vi "Create FPGA Addon.vi"(7 "group scalars":bool, 8 "error in":errorcluster, 10 "FPGA addon name":string, 11 "target in":refnum<k39>) -> (0 "error out":errorcluster, 2 "FPGA addon refnum":T1=18446744073709551615 format="%.0x", 3 "target out":refnum<k39>)   [LabVIEW 2026, in "Scripting API.lvlib"]
doc: "Creates an FPGA addon custom device within the provided System Definition Target. The FPGA addon name must be unique, otherwise the VI will return an error. The VI returns the reference of the created custom device.\n\nIf set to \"True\", the \"group scalars\" option allows the custom device to organize the FPGA bitfile controls and indicators into a folder structure following the \".\" notation (i.e. control bitfile name -> \"Group.myControl\" becomes a system definition channel \"myControl\" in the \"Group\" section -> Group\\myControl)"
uses:
  Scripting API.lvlib
  C:/Users/Administrator/Desktop/Jatin/All DNC DLLs/NationalInstruments.VeriStand.SystemDefinitionAPI.dll
  Jatin/All DNC DLLs/NationalInstruments.VeriStand.SystemDefinitionAPI.dll
  <vilib>/NI VeriStand/Custom Device API/Custom Device Item Ref.ctl
  Addon/Addon Shared/Types/FG Action.ctl
  Addon/Addon Shared/Types/FPGA Settings.ctl
  Addon/Addon Shared/SubVIs/Constants.vi
  <vilib>/NI VeriStand/Custom Device API/NI VeriStand - Get Item Property.vi
  <vilib>/NI VeriStand/Custom Device API/Get Item Property (Path).vi
  <vilib>/NI VeriStand/Custom Device API/Get Item Property (String).vi
  <vilib>/NI VeriStand/Custom Device API/Get Item Property (Boolean).vi
  <vilib>/NI VeriStand/Custom Device API/NI VeriStand - Set Item Property.vi
  <vilib>/NI VeriStand/Custom Device API/Set Item Property (Path).vi
  <vilib>/NI VeriStand/Custom Device API/Set Item Property (String).vi
  <vilib>/NI VeriStand/Custom Device API/Set Item Property (Boolean).vi
  Addon/Addon Shared/FPGA Addon Shared.lvlib
  <vilib>/NI VeriStand/Custom Device API/Custom Device API.lvlib
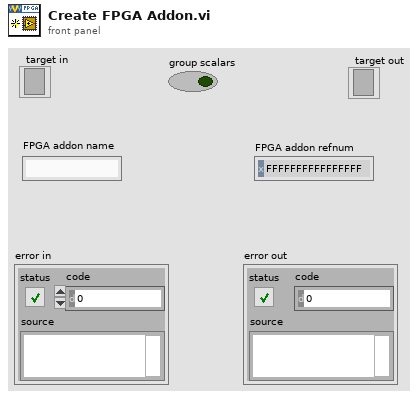
[diagram p1: front panel]
types:
  T1 = typedef "Custom Device API.lvlib/Custom Device Item Ref.ctl" = u64
  T2 = typedef "FPGA Addon Shared.lvlib/FPGA Settings.ctl" = cluster{"Bitfile path":path, "RIO Device Address":string, "Group":bool}
  T3 = typedef "FPGA Addon Shared.lvlib/FG Action.ctl" = enum8{"GET", "SET"}
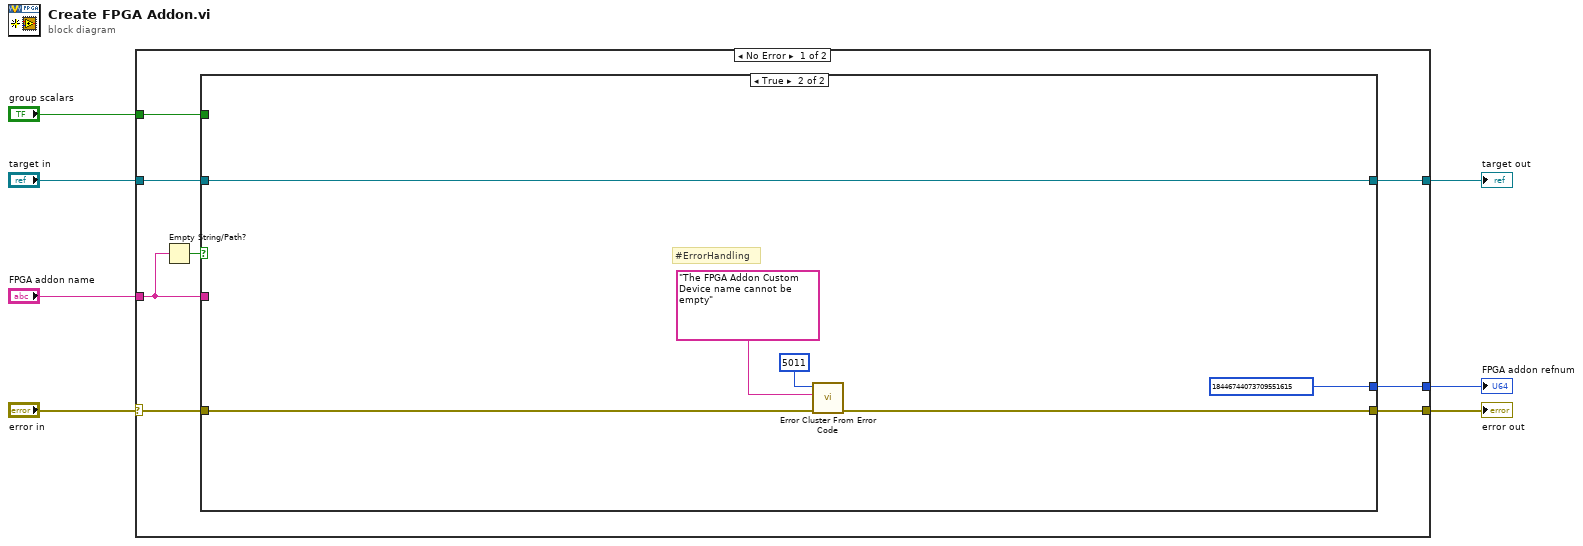
[diagram p0: block diagram]
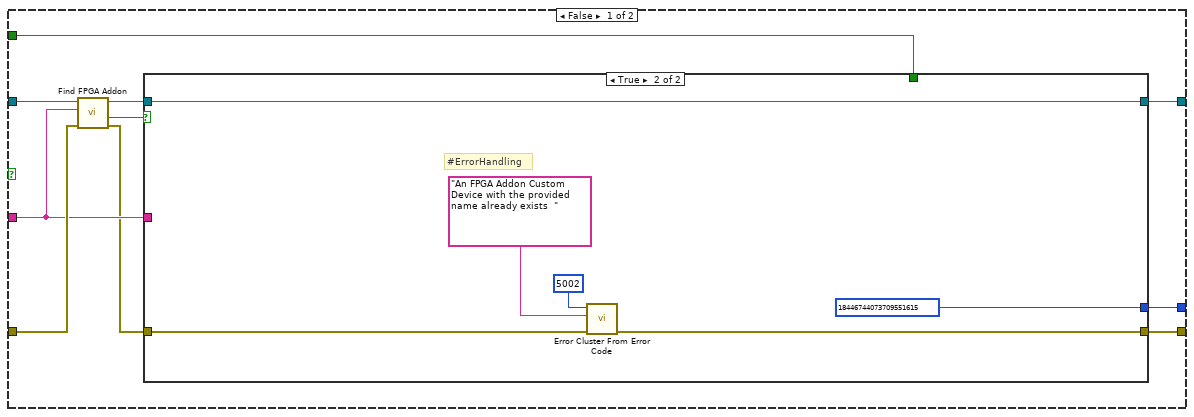
[diagram p2: hidden frame]
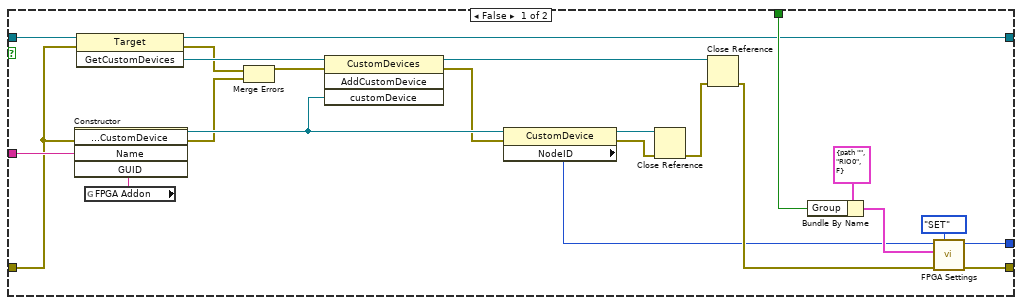
[diagram p3: hidden frame]
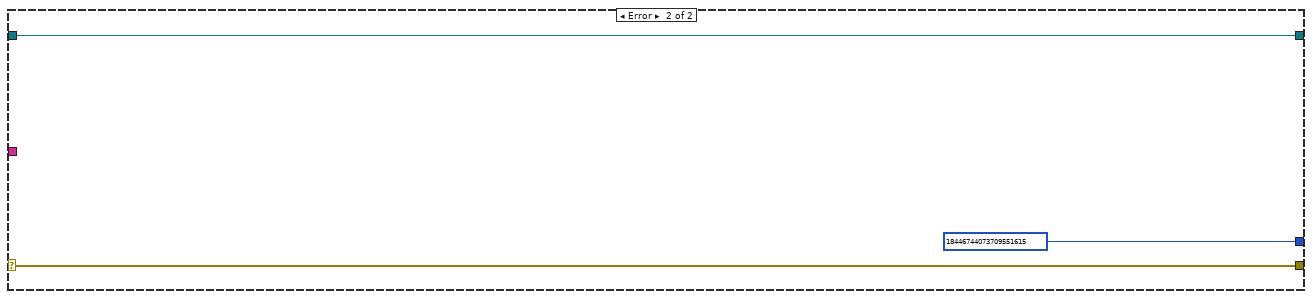
[diagram p4: hidden frame]
diagram:
  n1 = case shown="No Error" "error in" {
    selector: "error in" -> [w11 w61]
    tunnel: "target in" -> [w12 w63]
    tunnel: "FPGA addon name" -> [w8 _]
    tunnel: [w10 w63] -> w4
    tunnel: [w15 T1 18446744073709551615 ("FPGA Addon refnum")] -> w2
    tunnel: [w14 w61] -> w3
    tunnel: "group scalars" -> [w13 _]
    frame No Error {
      n2 = Empty String/Path?(string/path=w8) -> (empty?=w9:bool)
      n3 = case shown="True" w9 {
        tunnel: [w25 T1 18446744073709551615 ("FPGA Addon refnum")] -> w15
        tunnel: [w24 w57] -> w14
        tunnel: w13 -> [w23 _]
        tunnel: w12 -> [w22 w55]
        tunnel: w11 -> [w21 w58]
        tunnel: w8 -> [w20 _]
        tunnel: [w16 w55] -> w10
        frame False {
          n4 = call "Find FPGA Addon.vi"("error in"=w21, "FPGA addon name"=w20, "NationalInstruments.VeriStand.SystemDefinitionAPI.Target"=w22) -> ("error out"=w19:errorcluster, "found ?"=w18:bool, "NationalInstruments.VeriStand.SystemDefinitionAPI.Target"=w17:refnum<k39>)  [unwired: 5 in, 1 out]
          n5 = case shown="True" w18 {
            tunnel: [w35 T1 18446744073709551615 ("FPGA Addon refnum")] -> w25
            tunnel: [w34 w54] -> w24
            tunnel: w20 -> [w39 _]
            tunnel: w19 -> [w26 w50]
            tunnel: w23 -> [w31 _]
            tunnel: w17 -> [w30 w49]
            tunnel: [w29 w49] -> w16
            frame False {
              n6 = invoke class="Target" method="GetCustomDevices"(reference=w30, error in=w26) -> (reference out=w29:refnum<k39>, error out=w27:errorcluster, "GetCustomDevices"=w28:refnum<k39>)  [unwired: 1 in]
              n7 = global read "Constants.vi" "FPGA Addon"() -> (w47:string)
              n8 = constructor class="CustomDevice"(error in=w26, "Name"=w39, "GUID"=w47) -> (reference out=w48:refnum<k39>, error out=w46:errorcluster)  [unwired: 2 in, 3 out]
              n9 = Merge Errors(w27, w46) -> (w45:errorcluster)
              n10 = invoke class="CustomDevices" method="AddCustomDevice"(reference=w28, error in=w45, "customDevice"=w48) -> (reference out=w42:refnum<k39>, error out=w44:errorcluster)  [unwired: 1 in, 2 out]
              n11 = property class="CustomDevice"(reference=w48, error in=w44) -> (reference out=w40:refnum<k39>, error out=w43:errorcluster, "NodeID"=w32:u64)
              n12 = Close Reference(reference=w40, error in (no error)=w43) -> (error out=w41:errorcluster)
              n13 = Close Reference(reference=w42, error in (no error)=w41) -> (error out=w33:errorcluster)
              n14 = Bundle By Name(cluster=T2 {"Bitfile path"=path "", "RIO Device Address"="RIO0", "Group"=FALSE} ("FPGA Settings"), "Group"=w31) -> (w38:T2)
              n15 = call "FPGA Settings.vi"("Action"=FG_Action."SET", "error in (no error)"=w33, "FPGA Settings"=w38, "Item Ref"=w32) -> ("error out"=w34:errorcluster, "Item Ref out"=w35:T1)  [unwired: 5 in, 1 out]
            }
            frame True {
              # "#ErrorHandling"
              n16 = call <vilib>:"Error Cluster From Error Code.vi"("error in (no error)"=w50, "error message (\"\")"="An FPGA Addon Custom Device with the provided name already exists  " ("error message (\"\")"), "error code (0)"=5002) -> ("error out"=w54:errorcluster)  [unwired: 6 in]
            }
          }
        }
        frame True {
          # "#ErrorHandling"
          n17 = call <vilib>:"Error Cluster From Error Code.vi"("error in (no error)"=w58, "error message (\"\")"="The FPGA Addon Custom Device name cannot be empty" ("error message (\"\")"), "error code (0)"=5011) -> ("error out"=w57:errorcluster)  [unwired: 6 in]
        }
      }
    }
    frame Error {
    }
  }
  "target out" <- w4
  "error out" <- w3
  "FPGA addon refnum" <- w2
